vi "WildDrive_v2.vi"(9 "Super Turn":bool, 10 "Turn":dbl, 11 "Speed":dbl) -> (2 "Right Side Power":dbl, 3 "Left Side Power":dbl)   [LabVIEW 2018]
panel:
  in  "Manual Feed Forward (speed)":dbl=0.3
  in  "Manual Feed Forward (turn)":dbl=0.2
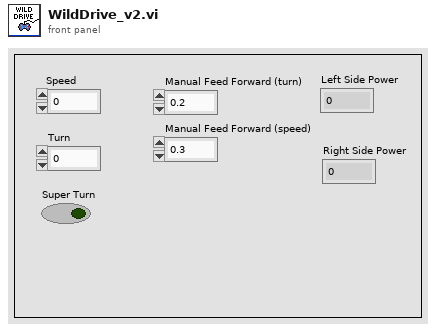
[diagram p1: front panel]
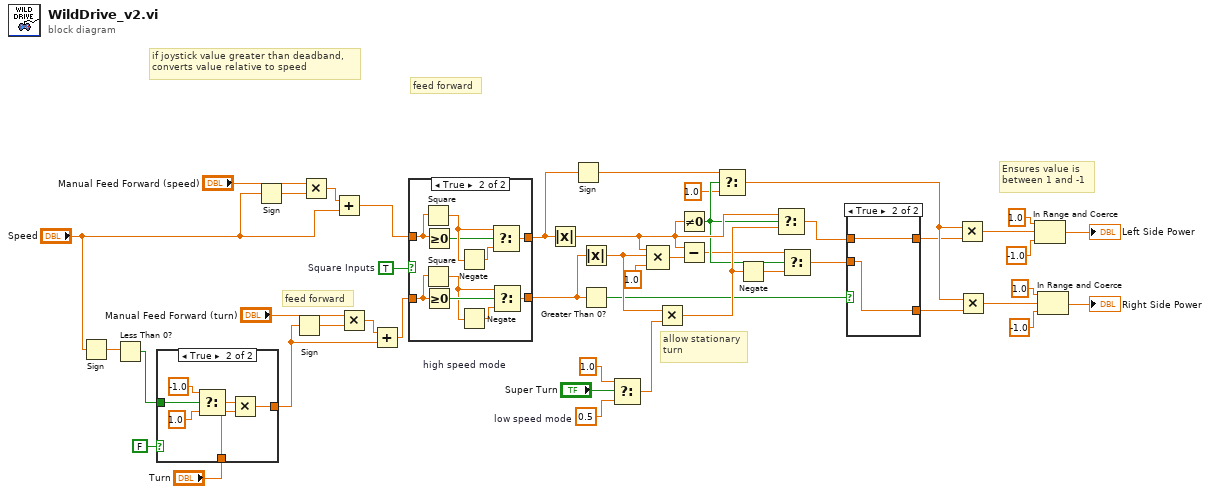
[diagram p0: block diagram]
diagram:
  w44 = 0.5  # low speed mode
  w43 = 1.0  # high speed mode
  w19 = TRUE  # Square Inputs
  # "feed forward"
  # "feed forward"
  # "Ensures value is \nbetween 1 and -1"
  # "if joystick value greater than deadband,\nconverts value relative to speed"
  # "allow stationary\nturn"
  n1 = Sign(1:"Speed") -> (0:w8:dbl)
  n2 = Less Than 0?(x=w8) -> (x < 0?=w10:bool)
  n3 = case shown="True" FALSE {
    tunnel: w10 -> [_ w51]
    tunnel: [w46 w48] -> w9
    tunnel: "Turn" -> [w46 w47]
    frame False {
    }
    frame True {
      n4 = Select(t=-1.0, s=w51, f=1.0) -> (s? t:f=w52:dbl)
      n5 = Multiply(x=w52, y=w47) -> (x*y=w48:dbl)
    }
  }
  n6 = Sign(1:"Speed") -> (0:w3:dbl)
  n7 = Sign(1:w9) -> (0:w11:dbl)
  n8 = Multiply(x="Manual Feed Forward (speed)", y=w3) -> (x*y=w4:dbl)
  n9 = Add(x=w4, y="Speed") -> (x+y=w1:dbl)
  n10 = Multiply(x="Manual Feed Forward (turn)", y=w11) -> (x*y=w12:dbl)
  n11 = Add(x=w12, y=w9) -> (x+y=w14:dbl)
  n12 = case shown="True" w19 {
    tunnel: [w53 w64] -> w16
    tunnel: [w54 w63] -> w15
    tunnel: w14 -> [w53 w62]
    tunnel: w1 -> [w54 w61]
    frame False {
    }
    frame True {
      n13 = Square(x=w61) -> (x^2=w56:dbl)
      n14 = Square(x=w62) -> (x^2=w59:dbl)
      n15 = Greater Or Equal To 0?(x=w61) -> (x >= 0?=w55:bool)
      n16 = Greater Or Equal To 0?(x=w62) -> (x >= 0?=w60:bool)
      n17 = Negate(x=w56) -> (-x=w57:dbl)
      n18 = Negate(x=w59) -> (-x=w58:dbl)
      n19 = Select(t=w56, s=w55, f=w57) -> (s? t:f=w63:dbl)
      n20 = Select(t=w59, s=w60, f=w58) -> (s? t:f=w64:dbl)
    }
  }
  n21 = Absolute Value(x=w15) -> (abs(x)=w28:dbl)
  n22 = Sign(1:w15) -> (0:w21:dbl)
  n23 = Absolute Value(x=w16) -> (abs(x)=w20:dbl)
  n24 = Greater Than 0?(x=w16) -> (x > 0?=w17:bool)
  n25 = Select(t=w43, s="Super Turn", f=w44) -> (s? t:f=w45:dbl)
  n26 = Compound Arithmetic op=MULTIPLY(w28, w20, 1.0 ("y")) -> (w23:dbl)
  n27 = Multiply(x=w20, y=w45) -> (x*y=w29:dbl)
  n28 = Not Equal To 0?(x=w28) -> (x != 0?=w27:bool)
  n29 = Subtract(x=w28, y=w23) -> (x-y=w25:dbl)
  n30 = Select(t=w21, s=w27, f=1.0) -> (s? t:f=w38:dbl)
  n31 = Negate(x=w29) -> (-x=w30:dbl)
  n32 = Select(t=w28, s=w27, f=w29) -> (s? t:f=w26:dbl)
  n33 = Select(t=w25, s=w27, f=w30) -> (s? t:f=w24:dbl)
  n34 = case shown="True" w17 {
    tunnel: w24 -> [w65 w68]
    tunnel: [w65 w67] -> w37
    tunnel: w26 -> [w66 w67]
    tunnel: [w66 w68] -> w39
    frame False {
    }
    frame True {
    }
  }
  n35 = Multiply(x=w38, y=w37) -> (x*y=w31:dbl)
  n36 = Multiply(x=w38, y=w39) -> (x*y=w36:dbl)
  n37 = In Range and Coerce(upper limit=1.0, x=w31, lower limit=-1.0) -> (coerced(x)=→"Left Side Power":dbl)  [unwired: 1 out]
  n38 = In Range and Coerce(upper limit=1.0, x=w36, lower limit=-1.0) -> (coerced(x)=→"Right Side Power":dbl)  [unwired: 1 out]
